vi "Write SLSC Switch Info.vi"(10 "Relays In":refnum<class "Relay.lvclass">[](array[class]), 11 "SLSC Switch in":refnum<class "SLSC Switch.lvclass">) -> (3 "SLSC Switch out":refnum<class "SLSC Switch.lvclass">)   [LabVIEW 2015, in "SLSC Switch.lvlib" / "SLSC Switch.lvclass"]
uses:
  SLSC Switch.lvclass
  Relay/Relay.lvclass
  SLSC Switch.lvclass/SLSC Switch.ctl
  Switch Action Processor/Switch Action Processor.lvclass
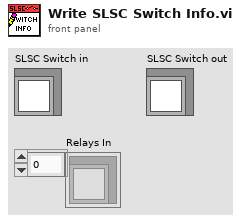
[diagram p1: front panel]
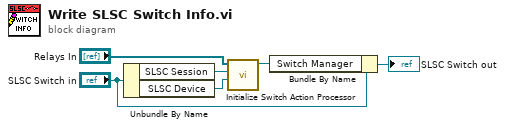
[diagram p0: block diagram]
diagram:
  n1 = Unbundle By Name("SLSC Switch in") -> ("SLSC Session"=w2:refnum<class "SLSC Interface.lvclass">, "SLSC Device"=w1:refnum<k21>)
  n2 = call "Initialize Switch Action Processor.vi"("SLSC Device"=w1, "SLSC Session in"=w2, "Relays"="Relays In") -> ("Switch Action Processor out"=w6:refnum<class "Switch Action Processor.lvclass">)  [unwired: 7 in, 1 out]
  n3 = Bundle By Name(cluster="SLSC Switch in", "Switch Manager"=w6) -> (→"SLSC Switch out":refnum<class "SLSC Switch.lvclass">)
